vi "Run.vi"(8 "error in (no error)":errorcluster caption="entrée d'erreur (pas d'erreur)", 9 "X":string[][](array[string]), 10 "Type X":T1(ring), 11 "normalize.lvclass":refnum<class "normalize.lvclass">) -> (0 "error out":errorcluster caption="sortie d'erreur", 2 "Data":T2, 3 "normalize.lvclass":refnum<class "normalize.lvclass">)   [LabVIEW 2020, in "normalize.lvclass"]
doc: "Returns : \n\n- X : {array-like, sparse matrix}, shape [n_samples, n_features]\nNormalized input X."
uses:
  normalize.lvclass
  normalize.lvclass/normalize.ctl
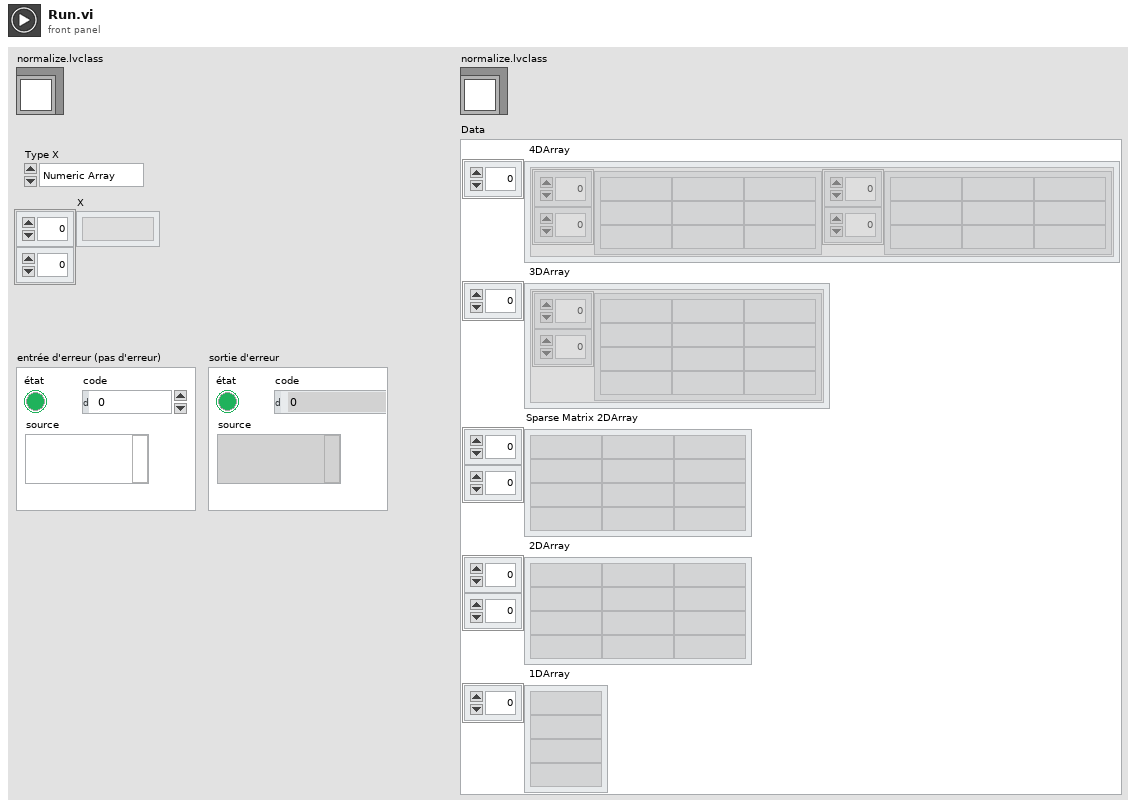
[diagram p1: front panel]
types:
  T1 = enum16{"Numeric Array", "String Array", "Sparse"}
  T2 = cluster{" 4DArray":cluster{"1":string[][], "2":string[][]}[], " 3DArray":cluster{"Tableau":string[][]}[], "Sparse Matrix 2DArray":string[][], " 2DArray":string[][], " 1DArray":string[]}
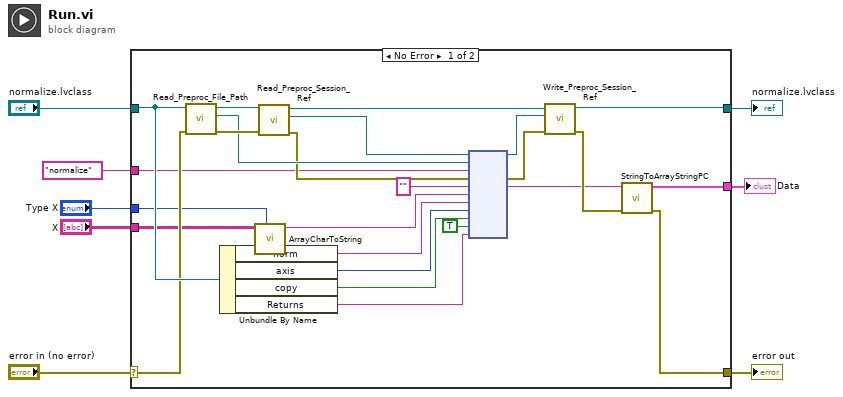
[diagram p0: block diagram]
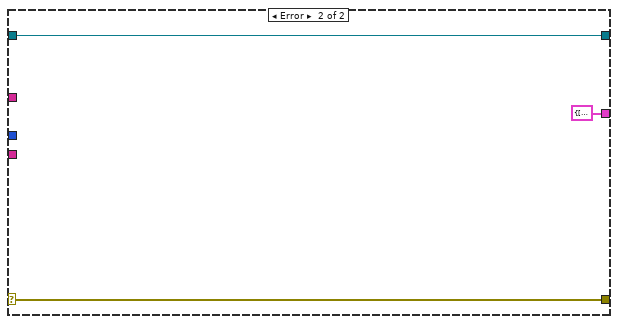
[diagram p2: hidden frame]
diagram:
  n1 = case shown="No Error" "error in (no error)" {
    selector: "error in (no error)" -> [w21 w36]
    tunnel: [w10 w36] -> w7
    tunnel: [w9 w35] -> w5
    tunnel: "normalize.lvclass" -> [w22 w35]
    tunnel: "normalize" ("Fonction") -> [w20 _]
    tunnel: [w11 T2 {" 4DArray"=[], " 3DArray"=[], "Sparse Matrix 2DArray"=[], " 2DArray"=[], " 1DArray"=[]} ("Data")] -> w1
    tunnel: "X" -> [w16 _]
    tunnel: "Type X" -> [w15 _]
    frame No Error {
      n2 = call-dynamic "Read_Preproc_File_Path.vi"("error in (no error)"=w21, "Python in"=w22) -> ("error out"=w32:errorcluster, "File_Path"=w29:path, "Python out"=w33:refnum<class "normalize.lvclass">)  [unwired: 7 in]
      n3 = Unbundle By Name(w22) -> ("norm"=w24:string, "axis"=w23:i32, "copy"=w19:bool, "Returns"=w17:string)
      n4 = call "ArrayCharToString.vi"("Type"=w15, "TAB"=w16) -> ("Instruction"=w14:string)  [unwired: 9 in]
      n5 = call-dynamic "Read_Preproc_Session_Ref.vi"("error in (no error)"=w32, "Python in"=w33) -> ("error out"=w28:errorcluster, "Session_ref"=w30:refnum<k35>, "Python out"=w31:refnum<class "normalize.lvclass">)  [unwired: 7 in]
      n6 = node(w30, w29, w20, w28, "", w14, w24, w23, w19, TRUE, w17) -> (w26:refnum<k35>, w27:errorcluster, w12:string)  [unwired: 6 in, 2 out]
      n7 = call-dynamic "Write_Preproc_Session_Ref.vi"("error in (no error)"=w27, "Session_ref"=w26, "Python in"=w31) -> ("error out"=w13:errorcluster, "Python out"=w9:refnum<class "normalize.lvclass">)  [unwired: 7 in]
      n8 = call "StringToArrayStringPC.vi"("sortie d'erreur"=w13, "Return value"=w12) -> ("sortie d'erreur"=w10:errorcluster, "Data"=w11:T2)  [unwired: 8 in]
    }
    frame Error {
    }
  }
  "error out" <- w7
  "normalize.lvclass" <- w5
  "Data" <- w1
